vi "arrays.vi"() -> ()   [LabVIEW 2020]
panel:
  out "Финал":i32[](array[numeric])
  out "Проверка":i32[](array[numeric])
  in  "Количество":dbl
  out "Массив рандома":dbl[](array[numeric])
  out "Округленный массив":i32[](array[numeric])
  in  "Диапазон":dbl
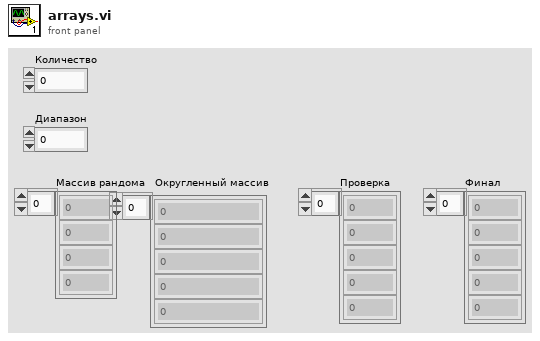
[diagram p1: front panel]
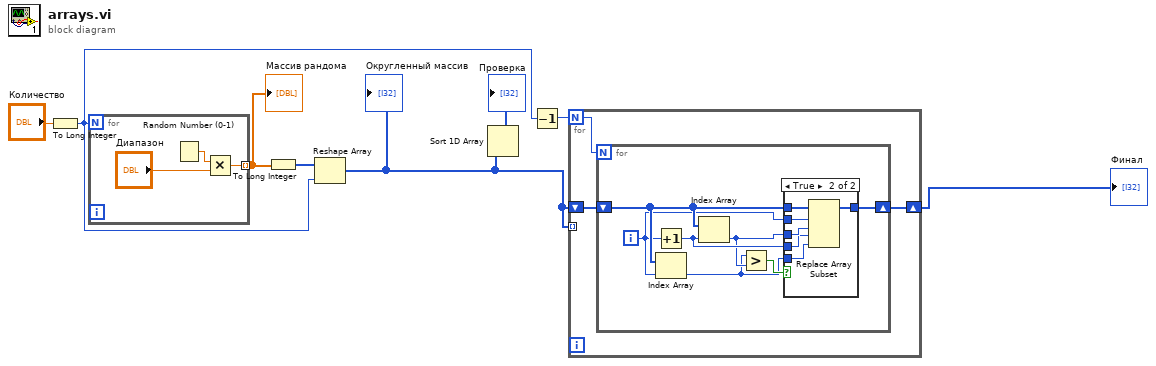
[diagram p0: block diagram]
diagram:
  n1 = To Long Integer(number="Количество") -> (32bit integer=w4:i32)
  n2 = for {
    N: w4 -> [_]
    tunnel: [w9] -> w6 mode=indexing
    n3 = Random Number (0-1)() -> (number: 0 to 1=w11:dbl)
    n4 = Multiply(x=w11, y="Диапазон") -> (x*y=w9:dbl)
  }
  "Массив рандома" <- w6
  n5 = To Long Integer(number=w6) -> (32bit integer=w8:i32[])
  n6 = Reshape Array(w8, w4) -> (w2:i32[])
  "Округленный массив" <- w2
  n7 = Sort 1D Array(array=w2) -> (sorted array=→"Проверка":i32[])
  n8 = Decrement(x=w4) -> (x-1=w3:i32)
  n9 = for {
    N: w3 -> [w14]
    tunnel: w2 -> [_] mode=indexing
    shift-right: [w12] -> w1
    shift-left: w2 -> [w13]
    n10 = for {
      N: w14 -> [_]
      shift-right: [w17] -> w12
      shift-left: w13 -> [w20]
      i -> [w19]
      n11 = Increment(x=w19) -> (x+1=w18:i32)
      n12 = Index Array(array=w20, index=w19) -> (element=w15:i32)
      n13 = Index Array(array=w20, index=w18) -> (element=w16:i32)
      n14 = Greater?(x=w15, y=w16) -> (0:w21:bool)
      n15 = case shown="True" w21 {
        tunnel: w20 -> [w22 w28]
        tunnel: w19 -> [_ w26]
        tunnel: w18 -> [_ w24]
        tunnel: [w22 w27] -> w17
        tunnel: w16 -> [_ w25]
        tunnel: w15 -> [_ w23]
        frame False {
        }
        frame True {
          n16 = Replace Array Subset(array=w28, new element #1=w25, index #1=w26, new element #2=w23, index #2=w24) -> (w27:i32[])
        }
      }
    }
  }
  "Финал" <- w1
